vi "Compare Class Types.vi"(1 "Class B":refnum<class>, 2 "Class A":refnum<class>) -> (0 "Class Types Equal?":bool)   [LabVIEW 2020, in "Utilities.lvlib"]
doc: "Compares class types. If the two objects are of the exact same class, this VI returns true, otherwise false."
uses:
  Utilities.lvlib
panel:
  out "error out":errorcluster
  in  "error in (no error)":errorcluster
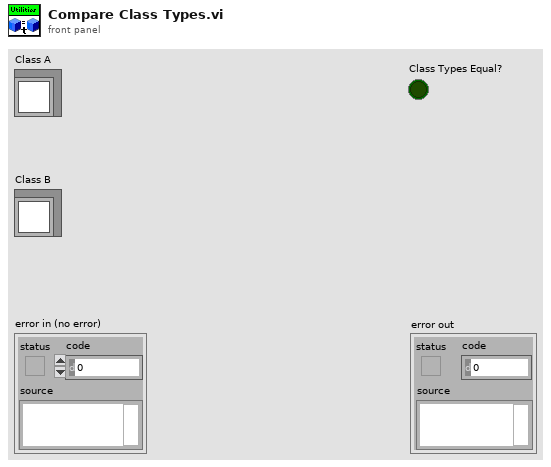
[diagram p1: front panel]
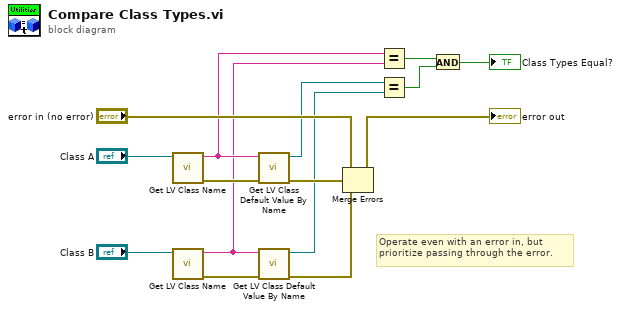
[diagram p0: block diagram]
diagram:
  # "Operate even with an error in, but prioritize passing through the error."
  n1 = call <vilib>:"Get LV Class Name.vi"("object"="Class A") -> ("error out"=w12:errorcluster, "class name"=w10:string)  [unwired: 9 in]
  n2 = call <vilib>:"Get LV Class Name.vi"("object"="Class B") -> ("error out"=w11:errorcluster, "class name"=w9:string)  [unwired: 9 in]
  n3 = call <vilib>:"Get LV Class Default Value By Name.vi"("error in (no error)"=w12, "class name"=w10) -> ("error out"=w8:errorcluster, "object"=w5:refnum<class>)  [unwired: 8 in]
  n4 = call <vilib>:"Get LV Class Default Value By Name.vi"("error in (no error)"=w11, "class name"=w9) -> ("error out"=w7:errorcluster, "object"=w4:refnum<class>)  [unwired: 8 in]
  n5 = Merge Errors("error in (no error)", w8, w7) -> (→"error out":errorcluster)
  n6 = Equal?(x=w10, y=w9) -> (x = y?=w3:bool)
  n7 = Equal?(x=w5, y=w4) -> (x = y?=w2:bool)
  n8 = And(x=w3, y=w2) -> (x .and. y?=→"Class Types Equal?":bool)
